vi "Write StationOptions.vi"(8 "error in (no error)":errorcluster, 10 "StationOptions":T8={"DataBase"={"Connection String Expression"="", "User ID"="", "Password"=""}, "Local Report"={"Report Path"=path "", "Report  Format"=enum."CSV", "Disabled State"=FALSE, "Customer name"=""}, "Localization"={"Language"=enum."English"}, "Preferences"={"Station ID"="", "IP Address"="", "Password"=""}, "  User Manager"={"Current User Manager File"="", "Login on start"=FALSE}, "Multiple UUT Settings"={"Number of Tests Sockets"=1, "Synchronization"=enum."Don't Synchronize"}, "Sequence"={"Sequence Folder Path"=path ""}} {"Multiple UUT Settings"."Number of Tests Sockets" min=1 step=1}, 11 "TestBench in":refnum<class "TestBench.lvclass">) -> (0 "error out":errorcluster, 3 "TestBench out":refnum<class "TestBench.lvclass">)   [LabVIEW 2019, in "TestBench.lvlib" / "TestBench.lvclass"]
uses:
  TestBench.lvclass
  SoftwareSetup/SoftwareSetup/DataBase.ctl
  SoftwareSetup/SoftwareSetup/Local Report.ctl
  SoftwareSetup/SoftwareSetup/Localization.ctl
  SoftwareSetup/SoftwareSetup/Preferences.ctl
  SoftwareSetup/SoftwareSetup/User Manager.ctl
  SoftwareSetup/SoftwareSetup/Multiple UUT Settings.ctl
  SoftwareSetup/SoftwareSetup/Sequence.ctl
  TestBench.lvclass/TestBench.ctl
  DataBase/DataBase Messages/RefreshTableName Msg/RefreshTableName Msg.lvclass/RefreshTableName Msg.ctl
  <vilib>/ActorFramework/Message Enqueuer/Message Enqueuer.lvclass/Message Enqueuer.ctl
  <vilib>/ActorFramework/Message Enqueuer/Enqueue.vi
  DataBase/DataBase Messages/RefreshTableName Msg/RefreshTableName Msg.lvclass
  C:/Program Files (x86)/National Instruments/LabVIEW 2019/vi.lib/ActorFramework/Message/Message.lvclass
  <vilib>/ActorFramework/Message Priority Queue/Priority Enqueue.vi
  SoftwareSetup/SoftwareSetup.lvlib
panel:
  # "Number of Tests Sockets"
  # "Synchronization"
  # "User Manager File"
  # "Station Info"
  # "MES Info"
  # "Select a Language:"
  # "Report File"
  # "Data Link Options"
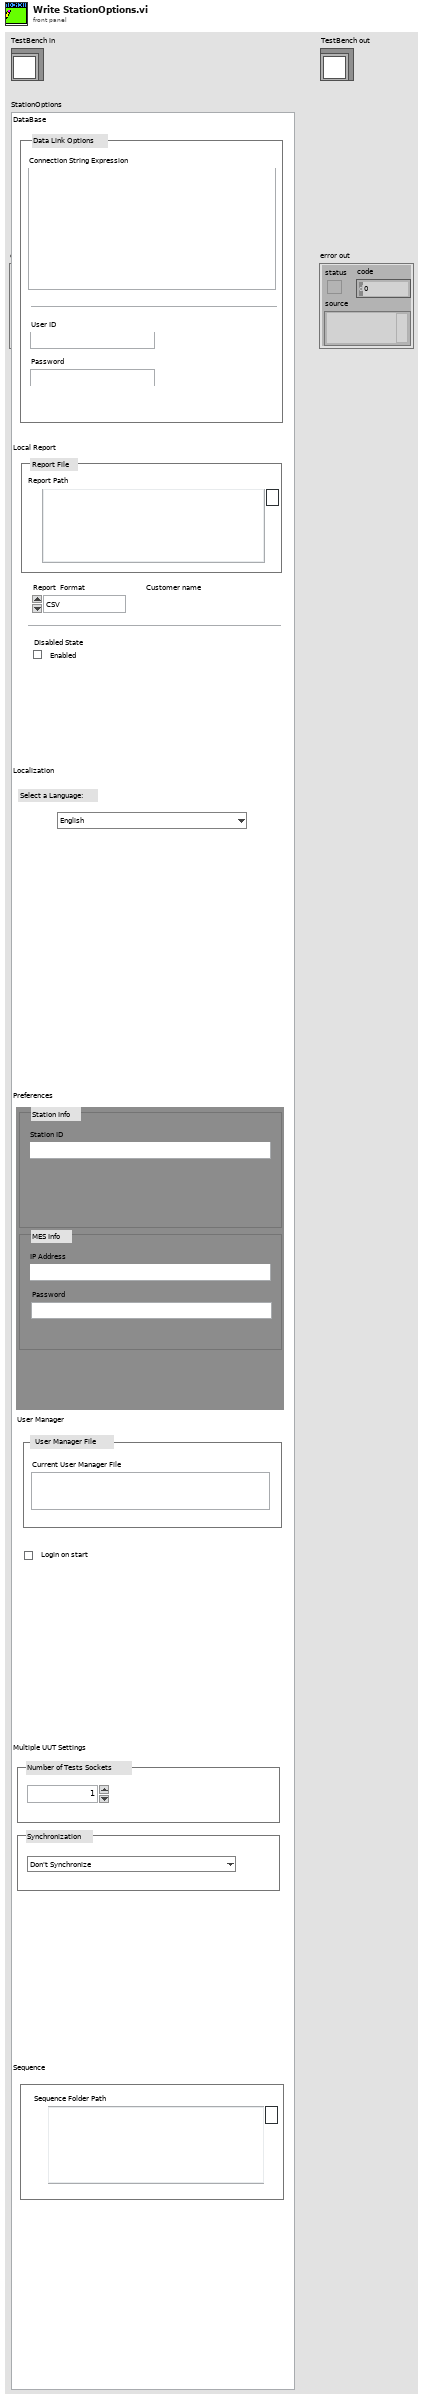
[diagram p1: front panel]
types:
  T1 = typedef "SoftwareSetup.lvlib/DataBase.ctl" = cluster{"Connection String Expression":string, "User ID":string, "Password":string}
  T2 = typedef "SoftwareSetup.lvlib/Local Report.ctl" = cluster{"Report Path":path, "Report  Format":enum16{"CSV", "XML", "PDF", "Excel", "TXT"}, "Disabled State":bool, "Customer name":string}
  T3 = typedef "SoftwareSetup.lvlib/Localization.ctl" = cluster{"Language":enum16{"English", "Chinese"}}
  T4 = typedef "SoftwareSetup.lvlib/Preferences.ctl" = cluster{"Station ID":string, "IP Address":string, "Password":string}
  T5 = typedef "SoftwareSetup.lvlib/User Manager.ctl" = cluster{"Current User Manager File":string, "Login on start":bool}
  T6 = typedef "SoftwareSetup.lvlib/Multiple UUT Settings.ctl" = cluster{"Number of Tests Sockets":u8, "Synchronization":enum16{"Don't Synchronize", "Serial", "Parallel", "One Thread Only"}}
  T7 = typedef "SoftwareSetup.lvlib/Sequence.ctl" = cluster{"Sequence Folder Path":path}
  T8 = cluster{"DataBase":T1, "Local Report":T2, "Localization":T3, "Preferences":T4, "  User Manager":T5, "Multiple UUT Settings":T6, "Sequence":T7}
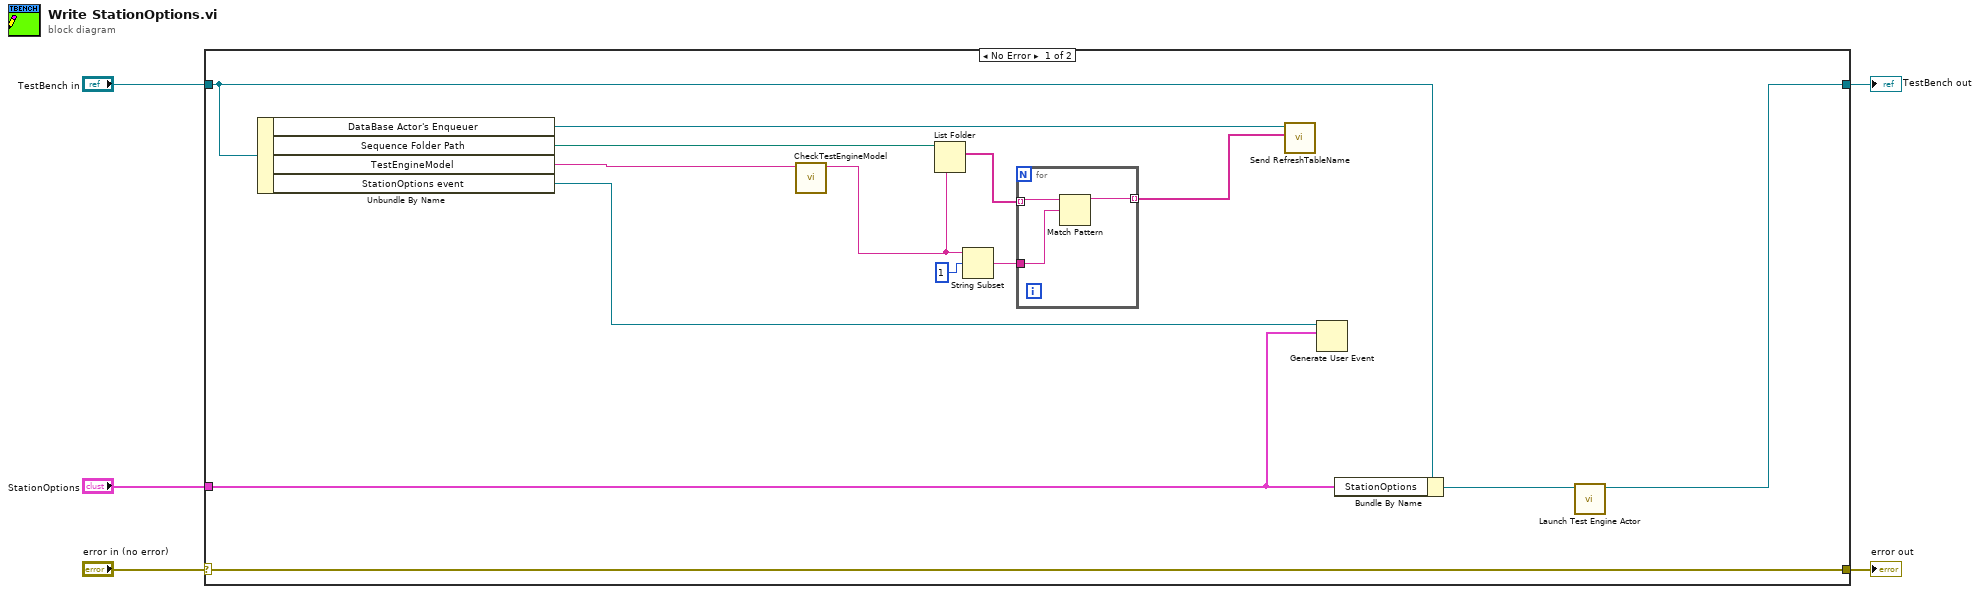
[diagram p0: block diagram]
diagram:
  n1 = case shown="No Error" "error in (no error)" {
    selector: "error in (no error)" -> [w19 w23]
    tunnel: [w19 w23] -> w4
    tunnel: [w6 w24] -> w2
    tunnel: "TestBench in" -> [w18 w24]
    tunnel: "StationOptions" -> [w16 _]
    frame No Error {
      n2 = Unbundle By Name(w18) -> ("DataBase Actor's Enqueuer"=w9:refnum<class "Message Enqueuer.lvclass">, "Sequence Folder Path"=w10:path, "TestEngineModel"=w11:string, "StationOptions event"=w17:refnum<user-event>)
      n3 = call "CheckTestEngineModel.vi"("Modle"=w11) -> ("Pattern"=w12:string)  [unwired: 10 in]
      n4 = List Folder(path=w10, pattern=w12) -> (filenames=w15:string[])  [unwired: 2 in, 3 out]
      n5 = String Subset(string=w12, offset (0)=1) -> (substring=w13:string)  [unwired: 1 in]
      n6 = for {
        tunnel: w15 -> [w22] mode=indexing
        tunnel: [w21] -> w8 mode=indexing
        tunnel: w13 -> [w20]
        n7 = Match Pattern(string=w22, regular expression=w20) -> (before substring=w21:string)  [unwired: 1 in, 3 out]
      }
      n8 = call "Send RefreshTableName.vi"("TableName"=w8, "Message Enqueuer"=w9) -> ()  [unwired: 8 in, 2 out]
      n9 = Generate User Event(user event=w17, event data cluster=w16) -> ()  [unwired: 2 in, 2 out]
      n10 = Bundle By Name(cluster=w18, "StationOptions"=w16) -> (w7:refnum<class "TestBench.lvclass">)
      n11 = call "Launch Test Engine Actor.vi"("TestBench in"=w7) -> ("TestBench out"=w6:refnum<class "TestBench.lvclass">)  [unwired: 9 in, 1 out]
    }
    frame Error {
    }
  }
  "error out" <- w4
  "TestBench out" <- w2
